vi "Set Ctrl Value.vi"(8 "error in (no error)":errorcluster, 10 "Variant":variant, 11 "Ctrl Refnum Column in":refnum<class "Ctrl Refnum Column.lvclass">) -> (0 "error out":errorcluster, 3 "Ctrl Refnum Column out":refnum<class "Ctrl Refnum Column.lvclass">)   [LabVIEW 2020, in "Basic Fields.lvlib" / "Ctrl Refnum Column.lvclass"]
uses:
  Ctrl Refnum Column.lvclass
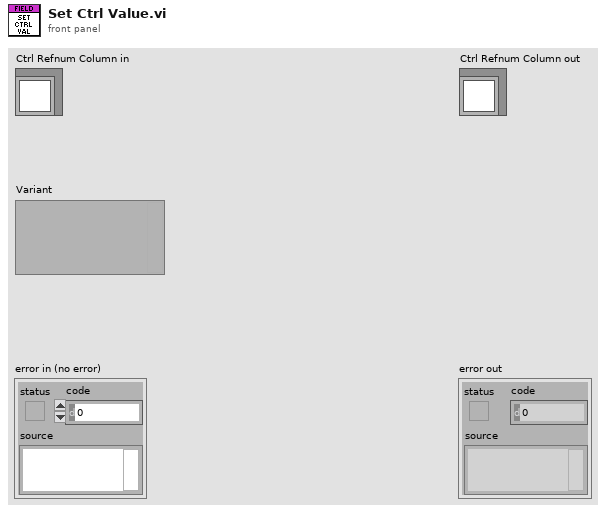
[diagram p1: front panel]
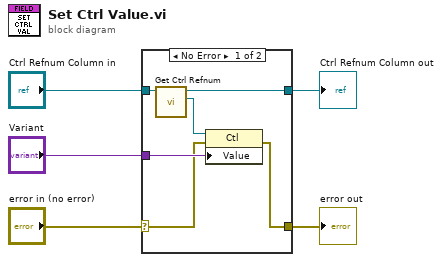
[diagram p0: block diagram]
diagram:
  n1 = case shown="No Error" "error in (no error)" {
    selector: "error in (no error)" -> [w7 w13]
    tunnel: [w6 w13] -> w4
    tunnel: [w10 w12] -> w2
    tunnel: "Ctrl Refnum Column in" -> [w11 w12]
    tunnel: "Variant" -> [w8 _]
    frame No Error {
      n2 = call-dynamic "Get Ctrl Refnum.vi"("Ctrl Refnum Column in"=w11) -> ("Ctl Refnum"=w9:refnum<vi>, "Ctrl Refnum Column out"=w10:refnum<class "Ctrl Refnum Column.lvclass">)  [unwired: 8 in, 1 out]
      n3 = property class="Ctl"(reference=w9, error in=w7, "Value"=w8) -> (error out=w6:errorcluster)  [unwired: 1 out]
    }
    frame Error {
    }
  }
  "error out" <- w4
  "Ctrl Refnum Column out" <- w2
